vi "SFOAE-Init Data File.vi"(0 "SFOAE":T3, 7 "State":T1) -> (4 "DataPath":path, 8 "Expt State out":T1)   [LabVIEW 2020]
uses:
  CFTS Main Panel SubVIs/CFTS-Experiment State.ctl
  Typedefs/SFOAE-Parameters.ctl
  Typedefs/SFOAE-Stimulus Parameters.ctl
  Typedefs/SFOAE-Sweep Params.ctl
  Typedefs/SFOAE-Response Parameters.ctl
  CFTS Main Panel SubVIs/CFTS-Data Type Enum.ctl
panel:
  out "error out":errorcluster
  in  "error in (no error)":errorcluster
  in  "Header":T2={"Data type"="SFOAE", "Filename"=path "", "Date"="", "Version"=0, "Heart Rate (/min)"=0.0, "Temp (C)"=0.0, "Notes"=""}
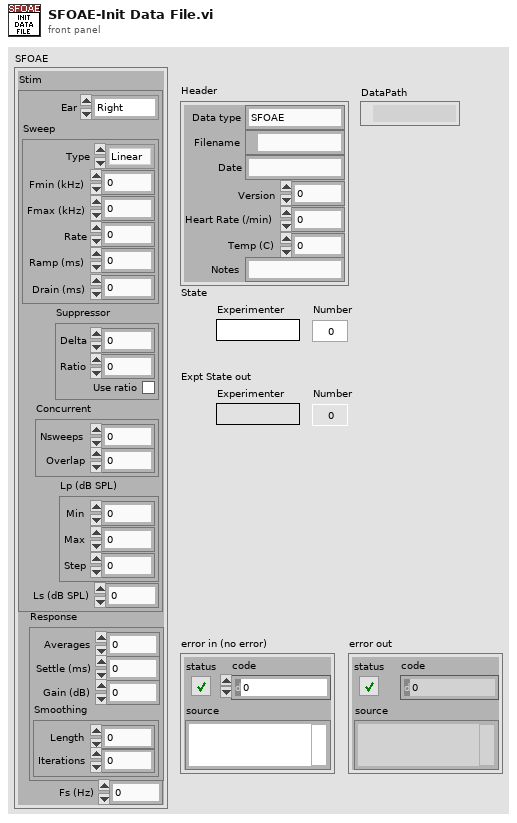
[diagram p1: front panel]
types:
  T1 = typedef "CFTS-Experiment State.ctl" = cluster{"Experimenter":string, "Number":u32, "Right":string, "Left":string, "Data Folder":path, "State File":path, "Version Info":string, "End Exposure Time":dbl, "Exposure Duration":string, "Run #":cluster{"CAP":i16, "ABR":i16, "DP":i16, "VsEP":i16, "MeasSeq":i16, "SubSeq":i16, "SFOAE":i16}}
  T2 = cluster{"Data type":string, "Filename":path, "Date":string, "Version":i32, "Heart Rate (/min)":dbl, "Temp (C)":dbl, "Notes":string}
  T3 = typedef "SFOAE-Parameters.ctl" = cluster{"Stim":T4, "Response":T6, "Fs (Hz)":dbl}
  T4 = typedef "SFOAE-Stimulus Parameters.ctl" = cluster{"Ear":enum16{"Right", "Left"}, "Sweep":T5, "Suppressor":cluster{"Delta":dbl, "Ratio":dbl, "Use ratio":bool}, "Concurrent":cluster{"Nsweeps":i32, "Overlap":dbl}, "Ls (dB SPL)":dbl, "Lp (dB SPL)":cluster{"Min":dbl, "Max":dbl, "Step":dbl}}
  T5 = typedef "SFOAE-Sweep Params.ctl" = cluster{"Type":enum16{"Linear", "Log"}, "Fmin (kHz)":dbl, "Fmax (kHz)":dbl, "Rate":dbl, "Ramp (ms)":dbl, "Drain (ms)":dbl}
  T6 = typedef "SFOAE-Response Parameters.ctl" = cluster{"Averages":i32, "Settle (ms)":dbl, "Gain (dB)":dbl, "Smoothing":cluster{"Length":i32, "Iterations":i32}}
  T7 = typedef "CFTS-Data Type Enum.ctl" = enum16{"CAP", "ABR", "DP", "VsEP", "MeasSeq", "SFOAE"}
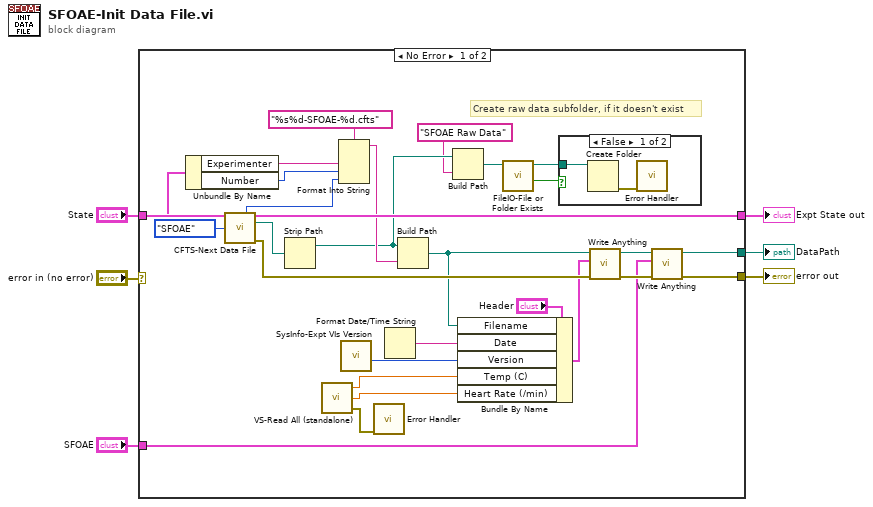
[diagram p0: block diagram]
diagram:
  n1 = case shown="No Error" "error in (no error)" {
    selector: "error in (no error)" -> [_ w37]
    tunnel: "SFOAE" -> [w23 _]
    tunnel: "State" -> [w28 w38]
    tunnel: [w20 w38] -> w3
    tunnel: [w22 w37] -> w2
    tunnel: [w8 _] -> w1
    frame No Error {
      # "Create raw data subfolder, if it doesn't exist"
      n2 = call "CFTS-Next Data File.vi"("Expt State"=w28, "Data Type"=CFTS-Data_Type_Enum."SFOAE") -> ("Run #"=w7:i16, "Expt State out"=w20:T1, "Datafile path"=w21:path, "error out"=w26:errorcluster)  [unwired: 9 in, 1 out]
      n3 = Unbundle By Name(w20) -> ("Experimenter"=w18:string, "Number"=w17:u32)
      n4 = Strip Path(path=w21) -> (stripped path=w14:path)  [unwired: 1 out]
      n5 = call "VS-Read All (standalone).vi"() -> ("error out"=w31:errorcluster, "Heart Rate (bpm)"=w29:dbl, "Temperature (C)"=w30:dbl)  [unwired: 3 in]
      n6 = Format Into String(format string="%s%d-SFOAE-%d.cfts", w18, w17, w7) -> (resulting string=w15:string)  [unwired: 2 in, 1 out]
      n7 = call "SysInfo-Expt VIs Version.vi"() -> ("Expt VIs Version out"=w32:i32)  [unwired: 11 in]
      n8 = call "Error Handler.vi"("error in (no error)"=w31) -> ()  [unwired: 13 in, 2 out]
      n9 = Format Date/Time String() -> (date/time string=w33:string)  [unwired: 3 in]
      n10 = Build Path(base path=w14, name or relative path=w15) -> (appended path=w16:path)
      n11 = Build Path(base path=w14, name or relative path="SFOAE Raw Data") -> (appended path=w12:path)
      n12 = Bundle By Name(cluster="Header", "Filename"=w16, "Date"=w33, "Version"=w32, "Temp (C)"=w30, "Heart Rate (/min)"=w29) -> (w25:T2)
      n13 = call "FileIO-File or Folder Exists.vi"("path"=w12) -> ("Exists?"=w11:bool, "dup path"=w10:path)  [unwired: 7 in, 2 out]
      n14 = case shown="False" w11 {
        tunnel: w10 -> [w36 _]
        frame False {
          n15 = Create Folder(path (use dialog)=w36) -> (error out=w35:errorcluster)  [unwired: 2 in, 2 out]
          n16 = call "Error Handler.vi"("error in (no error)"=w35) -> ()  [unwired: 13 in, 2 out]
        }
        frame True {
        }
      }
      n17 = call "Write Anything.vi"("Error In"=w26, "Anything"=w25, "Path (dialog)"=w16) -> ("Error Out"=w24:errorcluster, "Path out"=w9:path)  [unwired: 7 in]
      n18 = call "Write Anything.vi"("Error In"=w24, "Anything"=w23, "Path (dialog)"=w9) -> ("Error Out"=w22:errorcluster, "Path out"=w8:path)  [unwired: 7 in]
    }
    frame Error {
    }
  }
  "DataPath" <- w1
  "error out" <- w2
  "Expt State out" <- w3
